vi "WLAN_FrequencyOffsetEstimation(STF).vi"(10 "output cluster":cluster{"t0":dbl, "dt":dbl, "Y":cdb[]}) -> (2 "Frequency offset(STF)":dbl, 3 "output cluster 2":cluster{"t0":dbl, "dt":dbl, "Y":cdb[]})   [LabVIEW 2022 SP3]
uses:
  <vilib>/Analysis/baseanly.llb/Mean (DBL).vi
  <vilib>/Analysis/NI_AALBase.lvlib
panel:
  out "Waveform6":dbl[](graph)
  out "Waveform Graph":dbl[](graph)
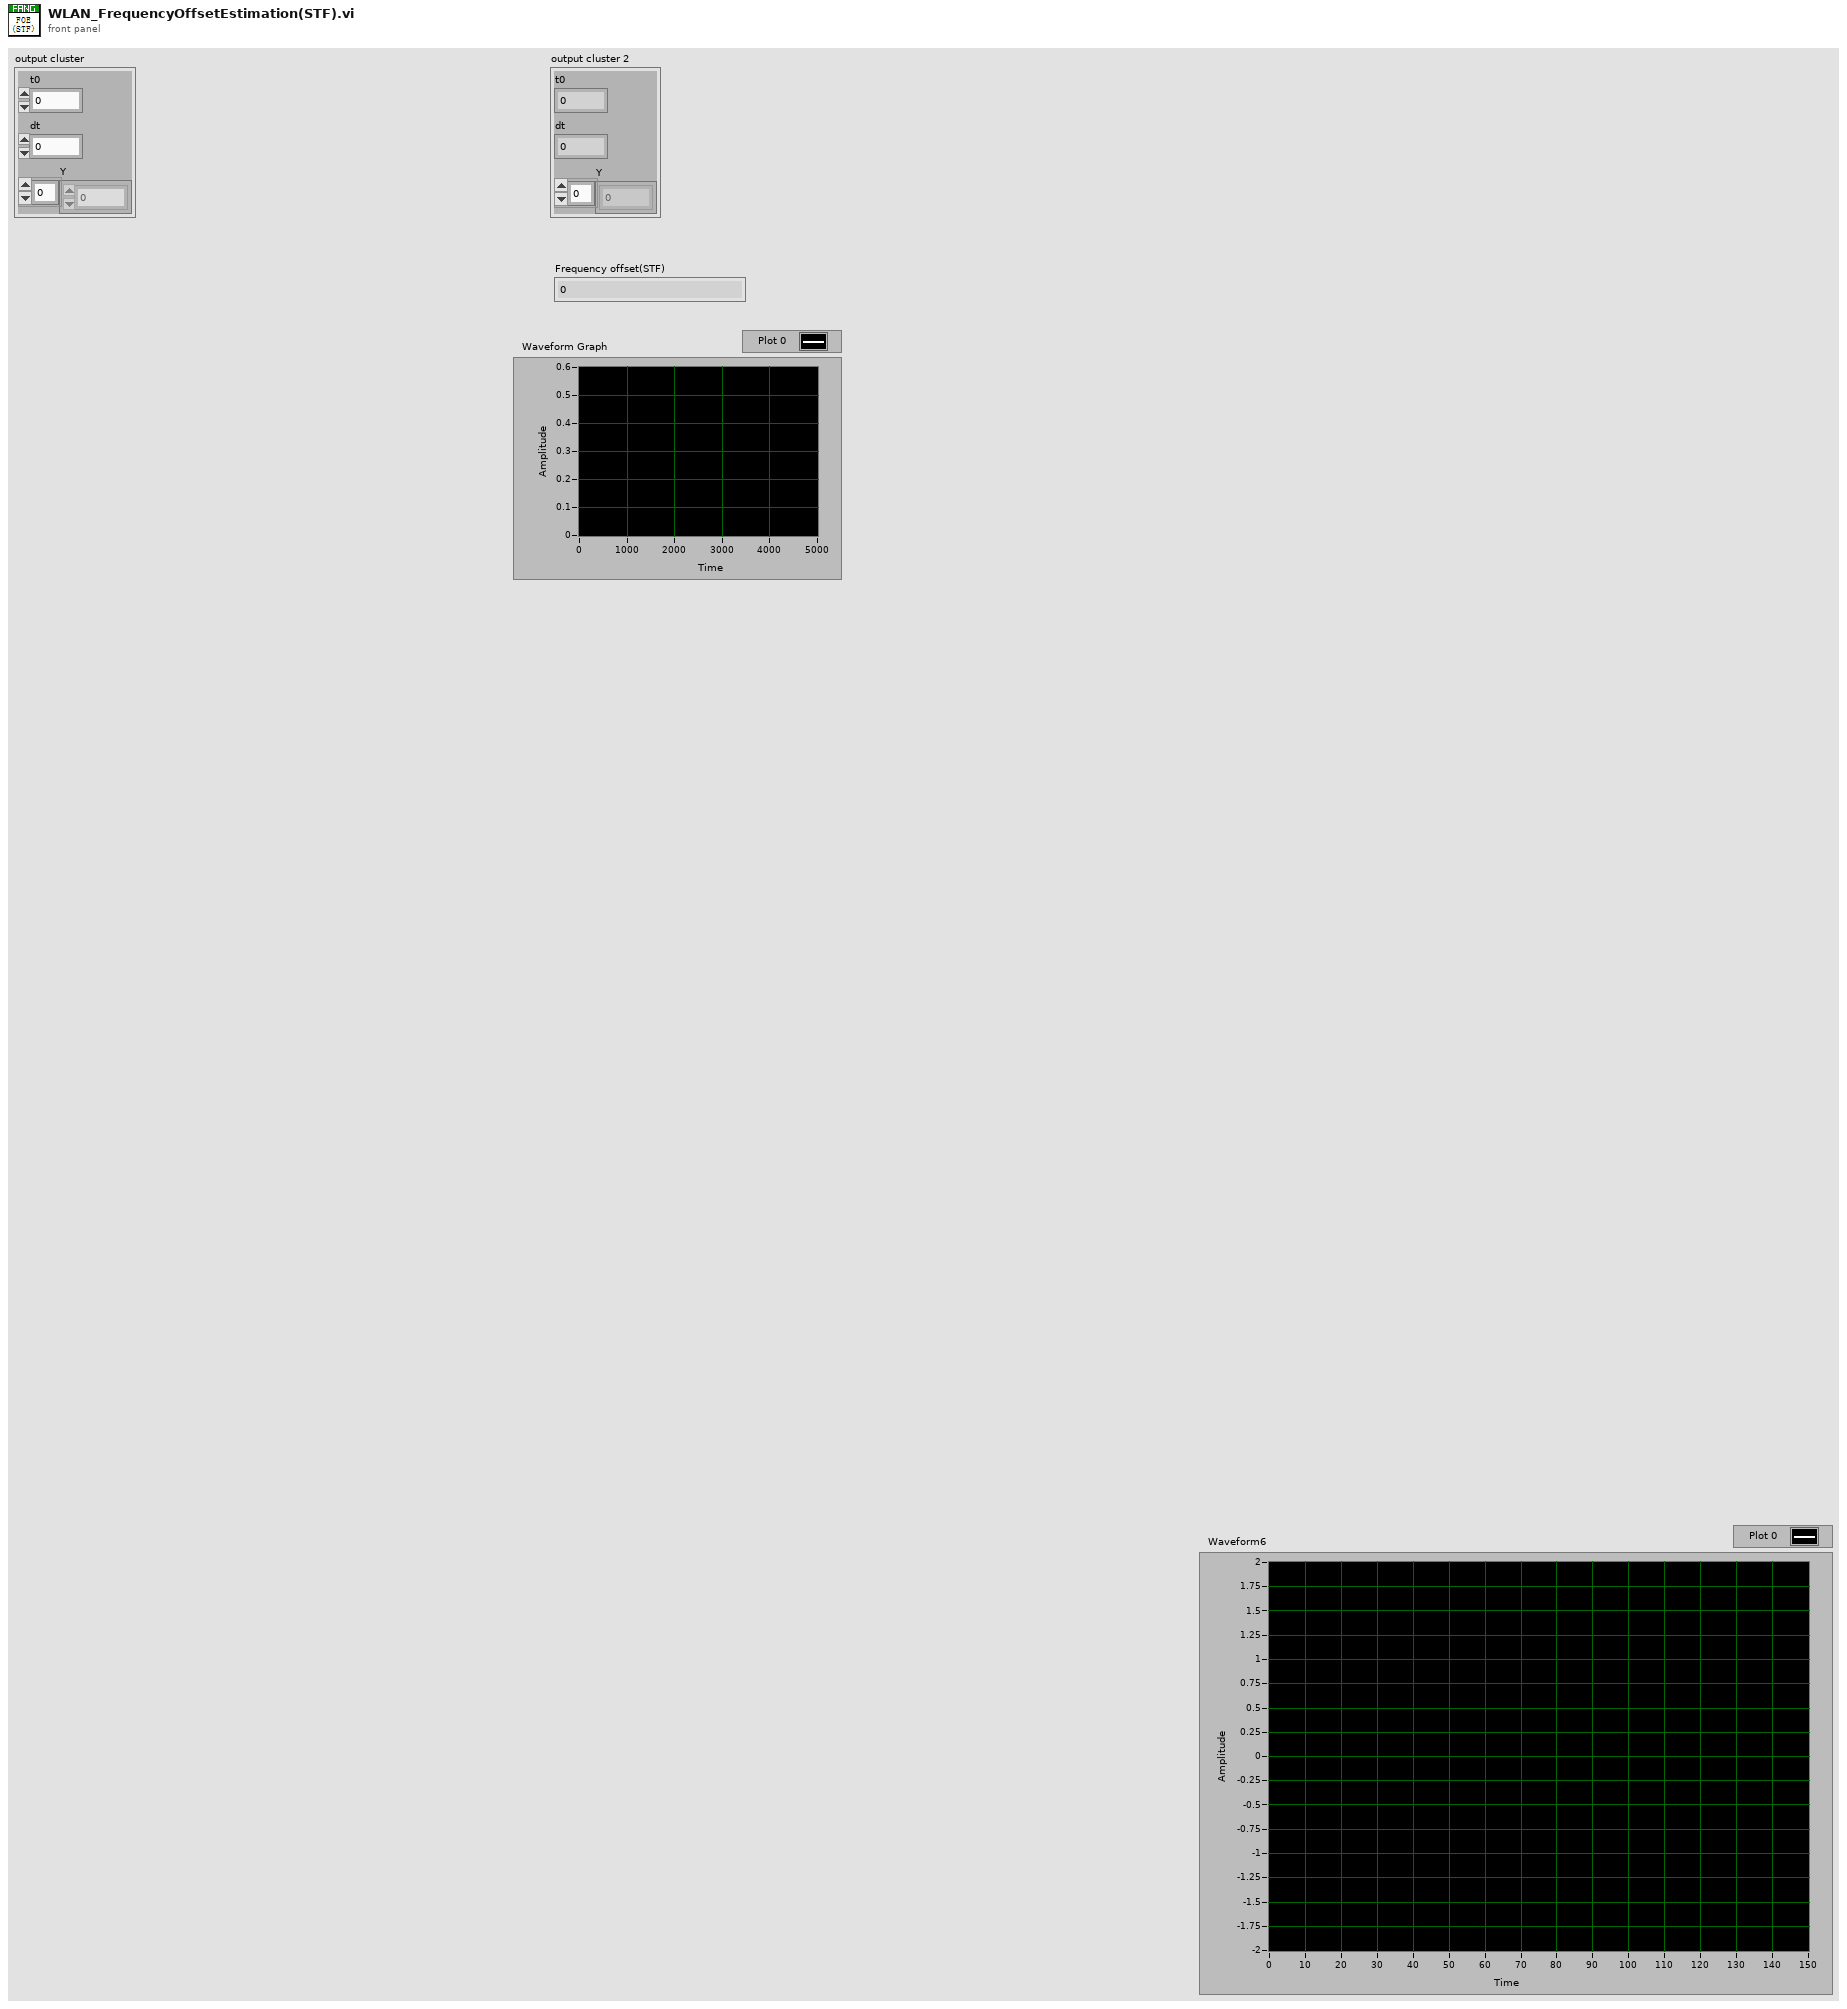
[diagram p1: front panel]
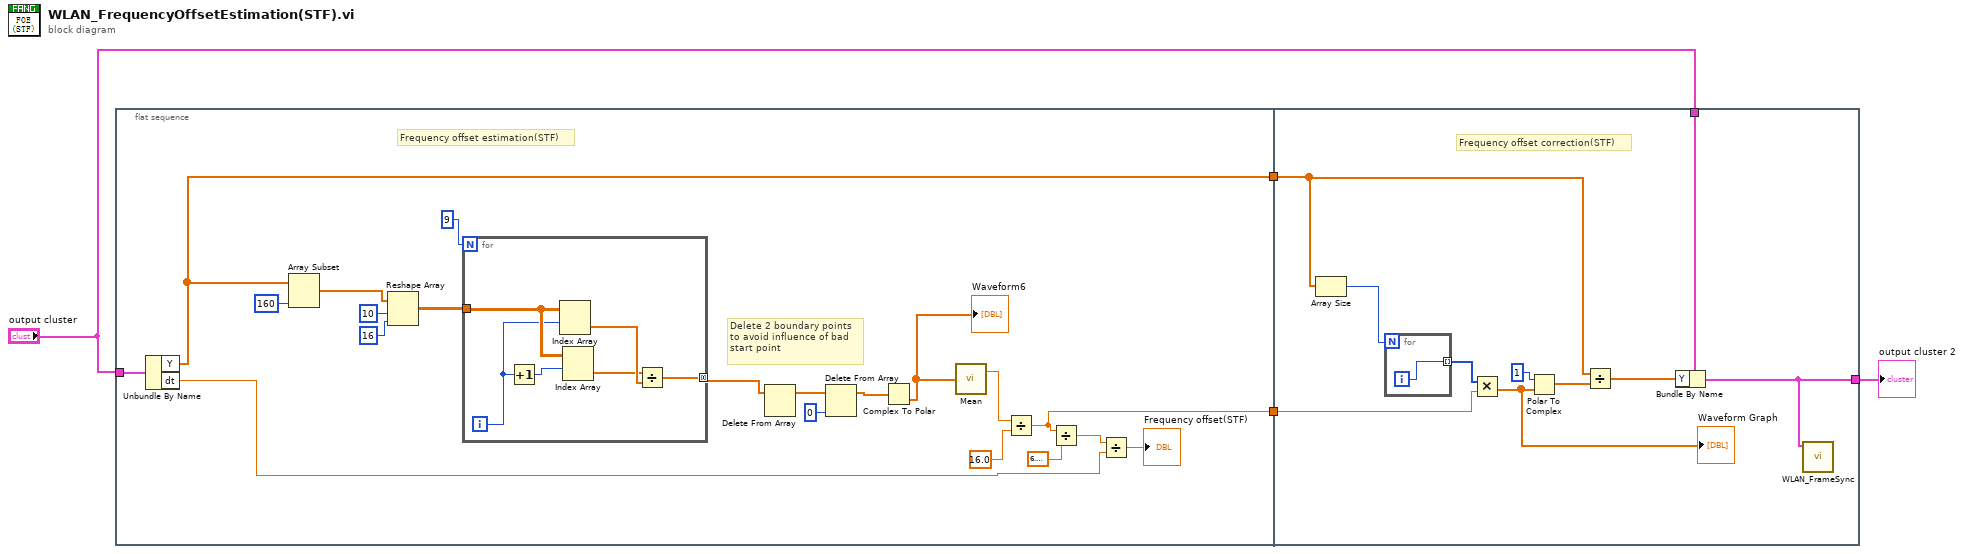
[diagram p0: block diagram]
diagram:
  n1 = flat-sequence {
    tunnel: "output cluster" -> [w12]
    tunnel: [w11] -> w4
    tunnel: [w10] -> w1
    tunnel: w4 -> [w34]
    tunnel: [w31] -> w3
    tunnel: "output cluster" -> [w33]
    tunnel: w1 -> [w32]
    frame #0 {
      # "Delete 2 boundary points\nto avoid influence of bad\nstart point"
      # "Frequency offset estimation(STF)"
      n2 = Unbundle By Name(w12) -> ("Y"=w11:cdb[], "dt"=w13:dbl)
      n3 = Array Subset(array=w11, length=160) -> (w24:cdb[])  [unwired: 1 in]
      n4 = Reshape Array(w24, 10 ("dimension size"), 16 ("dimension size")) -> (w22:cdb[][])
      n5 = for {
        N: 9 -> [_]
        tunnel: w22 -> [w30]
        tunnel: [w25] -> w8 mode=concatenating
        i -> [w28]
        n6 = Increment(x=w28) -> (x+1=w29:i32)
        n7 = Index Array(array=w30, index (row)=w28) -> (element=w27:cdb[])  [unwired: 1 in]
        n8 = Index Array(array=w30, index (row)=w29) -> (element=w26:cdb[])  [unwired: 1 in]
        n9 = Divide(x=w26, y=w27) -> (x/y=w25:cdb[])
      }
      n10 = Delete From Array(array=w8) -> (array with subset deleted=w7:cdb[])  [unwired: 2 in, 1 out]
      n11 = Delete From Array(array=w7, index=0) -> (array with subset deleted=w6:cdb[])  [unwired: 1 in, 1 out]
      n12 = Complex To Polar(r * e^(i*theta)=w6) -> (theta=w9:dbl[])  [unwired: 1 out]
      "Waveform6" <- w9
      n13 = call-poly <vilib>:"Mean.vi"("X"=w9) -> ("mean"=w14:dbl)  [unwired: 1 out]
      n14 = Divide(x=w14, y=16.0) -> (x/y=w10:dbl)
      n15 = Divide(x=w10, y=6.283185307179586) -> (x/y=w16:dbl)
      n16 = Divide(x=w16, y=w13) -> (x/y=→"Frequency offset(STF)":dbl)
    }
    frame #1 {
      # "Frequency offset correction(STF)"
      n17 = Array Size(array=w34) -> (size(s)=w36:i32)
      n18 = for {
        N: w36 -> [_]
        tunnel: [w41] -> w35 mode=indexing
        i -> [w41]
      }
      n19 = Multiply(x=w35, y=w32) -> (x*y=w40:dbl[])
      "Waveform Graph" <- w40
      n20 = Polar To Complex(1:w40, 2:1) -> (0:w38:cdb[])
      n21 = Divide(x=w34, y=w38) -> (x/y=w39:cdb[])
      n22 = Bundle By Name(cluster=w33, "Y"=w39) -> (w31:cluster{"t0":dbl, "dt":dbl, "Y":cdb[]})
      n23 = call "WLAN_FrameSync.vi"("input cluster"=w31) -> ()  [unwired: 9 in, 2 out]
    }
  }
  "output cluster 2" <- w3
